vi "Create Session Reservation.vi"(7 "reservation observer":refnum<class "IReservation Observer.lvclass">, 8 "error in":errorcluster, 9 "session reservation response":T1, 10 "pin or relay names":string[](array[string]), 11 "pin map context":T8) -> (0 "error out":errorcluster, 3 "session reservation out":refnum<class "Session Reservation.lvclass">)   [LabVIEW 2020, in "Measurement Plugin Session Management V1.lvlib" / "Session Reservation.lvclass"]
doc: "Collects all the session reservation related data and creates a session reservation data value reference of the session reservation class."
uses:
  Session Reservation.lvclass
  gRPC/Generated APIs/ni/measurementlink/sessionmanagement/v1/RPC Messages/ni_measurementlink_PinMapContext.ctl
  IReservation Observer/IReservation Observer.lvclass
  gRPC/Generated APIs/ni/measurementlink/sessionmanagement/v1/RPC Messages/ni_measurementlink_sessionmanagement_v1_ReserveSessionsResponse.ctl
  gRPC/Generated APIs/ni/measurementlink/sessionmanagement/v1/RPC Messages/ni_measurementlink_sessionmanagement_v1_SessionInformation.ctl
  gRPC/Generated APIs/ni/measurementlink/sessionmanagement/v1/RPC Messages/nidevice_grpc_Session.ctl
  gRPC/Generated APIs/ni/measurementlink/sessionmanagement/v1/RPC Messages/ni_measurementlink_sessionmanagement_v1_ChannelMapping.ctl
  gRPC/Generated APIs/ni/measurementlink/sessionmanagement/v1/RPC Messages/ni_measurementlink_sessionmanagement_v1_MultiplexerSessionInformation.ctl
  gRPC/Generated APIs/ni/measurementlink/sessionmanagement/v1/RPC Messages/ni_measurementlink_sessionmanagement_v1_ReserveSessionsResponse_GroupMappingsEntry.ctl
  gRPC/Generated APIs/ni/measurementlink/sessionmanagement/v1/RPC Messages/ni_measurementlink_sessionmanagement_v1_ResolvedPinsOrRelays.ctl
  Data.ctl
  Session and Driver Info.ctl
  Sessions/Instrument Sessions/ISession Factory/ISession Factory.lvclass
  Sessions/Instrument Sessions/ISession Factory/Initialize and Close Session Behavior.ctl
  Connection Map/Connection Map.lvclass
  Group Mapping.ctl
  <vilib>/Utility/miscctls.llb/LVMapReplaceAction.ctl
  Session Reservation.lvclass/Session Reservation.ctl
  gRPC/Generated APIs/ni/measurementlink/sessionmanagement/v1/ni.measurementlink.sessionmanagement.v1.lvlib
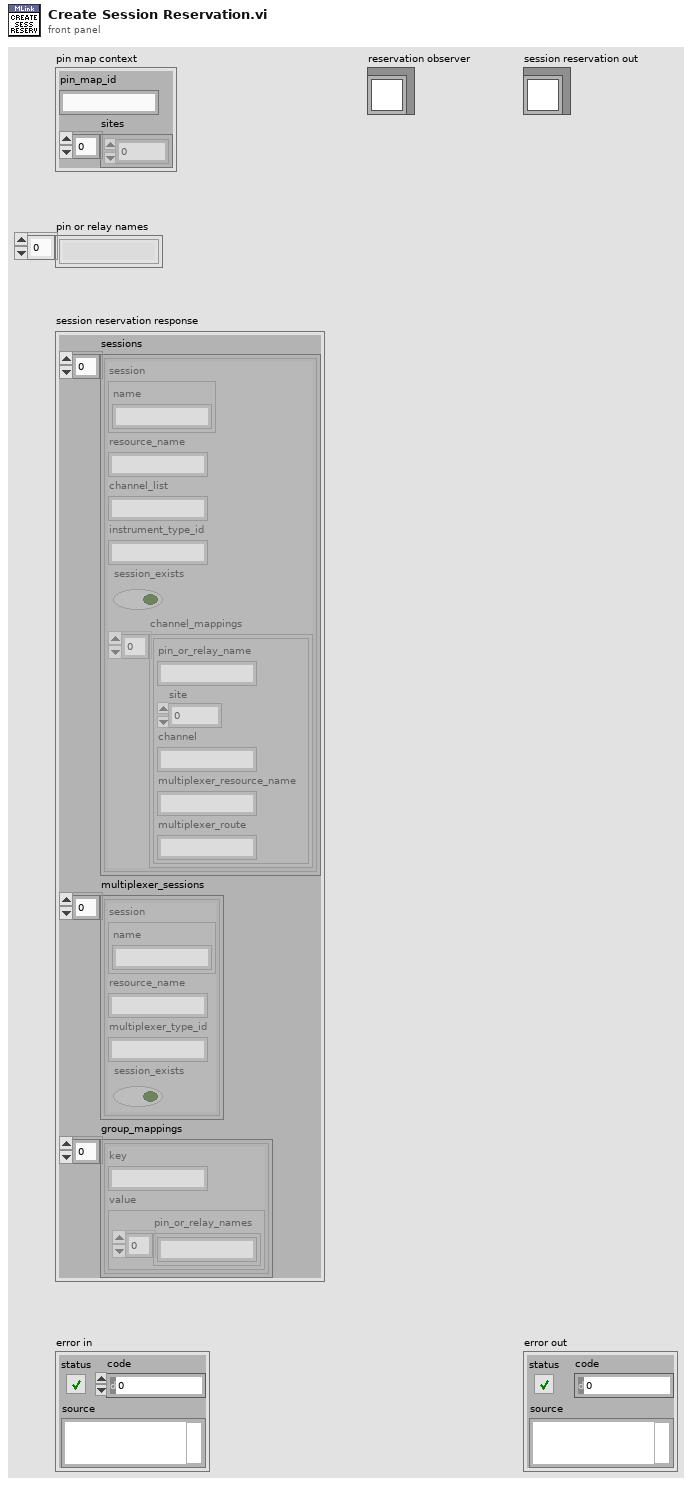
[diagram p1: front panel]
types:
  T1 = typedef "ni.measurementlink.sessionmanagement.v1.lvlib/ni_measurementlink_sessionmanagement_v1_ReserveSessionsResponse.ctl" = cluster{"sessions":T2[], "multiplexer_sessions":T5[], "group_mappings":T6[]}
  T2 = typedef "ni.measurementlink.sessionmanagement.v1.lvlib/ni_measurementlink_sessionmanagement_v1_SessionInformation.ctl" = cluster{"session":T3, "resource_name":string, "channel_list":string, "instrument_type_id":string, "session_exists":bool, "channel_mappings":T4[]}
  T3 = typedef "ni.measurementlink.sessionmanagement.v1.lvlib/nidevice_grpc_Session.ctl" = cluster{"name":string}
  T4 = typedef "ni.measurementlink.sessionmanagement.v1.lvlib/ni_measurementlink_sessionmanagement_v1_ChannelMapping.ctl" = cluster{"pin_or_relay_name":string, "site":i32, "channel":string, "multiplexer_resource_name":string, "multiplexer_route":string}
  T5 = typedef "ni.measurementlink.sessionmanagement.v1.lvlib/ni_measurementlink_sessionmanagement_v1_MultiplexerSessionInformation.ctl" = cluster{"session":T3, "resource_name":string, "multiplexer_type_id":string, "session_exists":bool}
  T6 = typedef "ni.measurementlink.sessionmanagement.v1.lvlib/ni_measurementlink_sessionmanagement_v1_ReserveSessionsResponse_GroupMappingsEntry.ctl" = cluster{"key":string, "value":T7}
  T7 = typedef "ni.measurementlink.sessionmanagement.v1.lvlib/ni_measurementlink_sessionmanagement_v1_ResolvedPinsOrRelays.ctl" = cluster{"pin_or_relay_names":string[]}
  T8 = typedef "ni.measurementlink.sessionmanagement.v1.lvlib/ni_measurementlink_PinMapContext.ctl" = cluster{"pin_map_id":string, "sites":i32[]}
  T9 = typedef "Measurement Plugin Session Management V1.lvlib/Session Reservation.lvclass/Data.ctl" = cluster{"session and driver infos":T10[], "pin or relay names":string[], "connection map":refnum<class "Connection Map.lvclass">, "pin map context":T8, "reservation observer":refnum<class "IReservation Observer.lvclass">, "dvr valid":bool, "group mappings":T12}
  T10 = typedef "Measurement Plugin Session Management V1.lvlib/Session Reservation.lvclass/Session and Driver Info.ctl" = cluster{"session info":T2, "session":variant, "session factory":refnum<class "ISession Factory.lvclass">, "initialize and close session behavior":T11}
  T11 = typedef "Instrument Sessions.lvlib/ISession Factory.lvclass/Initialize and Close Session Behavior.ctl" = enum16{"Initialize and Close", "Attach and Detach", "Initialize and Detach", "Attach and Close"}
  T12 = typedef "Measurement Plugin Session Management V1.lvlib/Session Reservation.lvclass/Group Mapping.ctl" = map{string, string[]}
  T13 = typedef "LVMapReplaceAction.ctl" = enum32{"Modify Entry only if found", "Add or Modify Entry", "Delete Entry"}
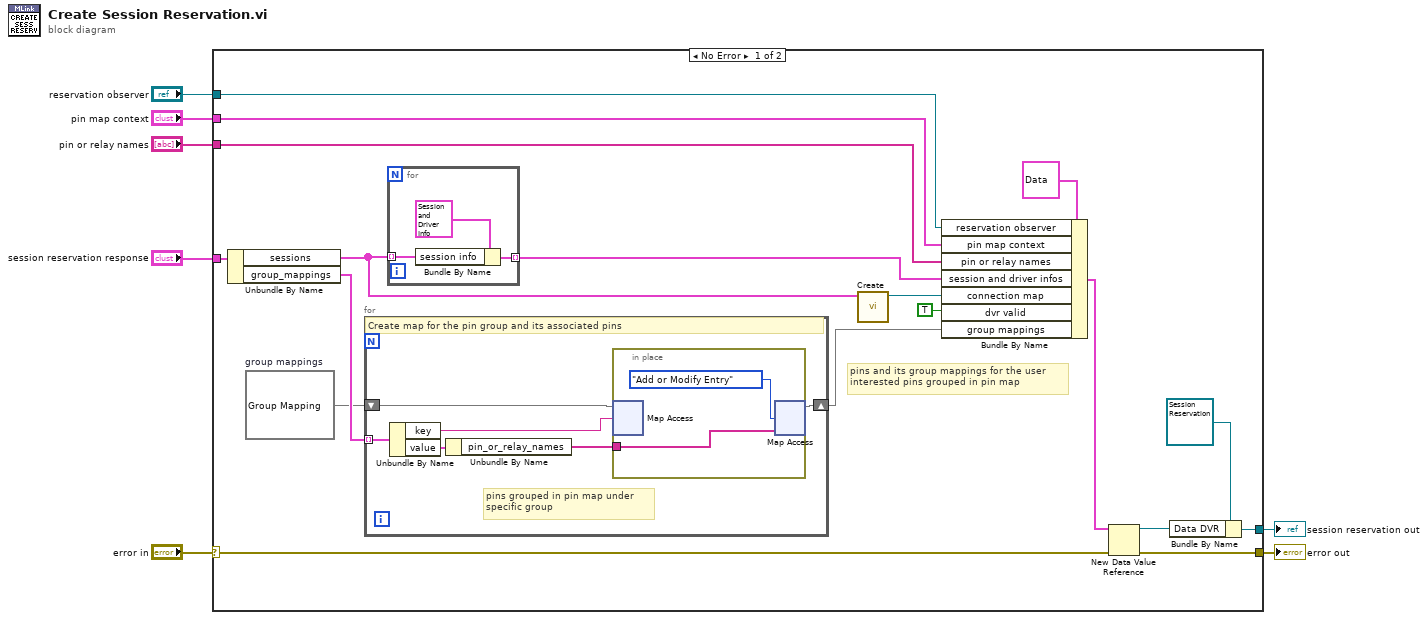
[diagram p0: block diagram]
diagram:
  n1 = case shown="No Error" "error in" {
    selector: "error in" -> [w15 w37]
    tunnel: [w19 w37] -> w7
    tunnel: [w18 _] -> w6
    tunnel: "pin map context" -> [w17 _]
    tunnel: "pin or relay names" -> [w16 _]
    tunnel: "reservation observer" -> [w14 _]
    tunnel: "session reservation response" -> [w12 _]
    frame No Error {
      w9 = T12 {}  # group mappings
      # "pins and its group mappings for the user \ninterested pins grouped in pin map"
      n2 = Unbundle By Name(w12) -> ("sessions"=w11:T2[], "group_mappings"=w10:T6[])
      n3 = for {
        tunnel: w10 -> [w31] mode=indexing
        shift-right: [w29] -> w8
        shift-left: w9 -> [w28]
        # "pins grouped in pin map under \nspecific group"
        # "Create map for the pin group and its associated pins"
        n4 = Unbundle By Name(w31) -> ("key"=w27:string, "value"=w30:T7)
        n5 = Unbundle By Name(w30) -> ("pin_or_relay_names"=w26:string[])
        n6 = in-place {
          in-place-border: w26 -> [w32]
          n7 = in-place-map #1(w28, w27) -> ()  [unwired: 1 in, 2 out]
          n8 = in-place-map #1(w32, LVMapReplaceAction."Add or Modify Entry" ("action")) -> (w29:T12)  [unwired: 2 out]
        }
      }
      n9 = for {
        tunnel: w11 -> [w36] mode=indexing
        tunnel: [w35] -> w25 mode=indexing
        n10 = Bundle By Name(cluster=T10 {"session info"={"session"={"name"=""}, "resource_name"="", "channel_list"="", "instrument_type_id"="", "session_exists"=FALSE, "channel_mappings"=[]}, "session"=variant, "session factory"=refnum, "initialize and close session behavior"=enum."Initialize and Close"} ("session and driver info"), "session info"=w36) -> (w35:T10)
      }
      n11 = call "Create.vi"("session info"=w11) -> ("connection map"=w24:refnum<class "Connection Map.lvclass">)  [unwired: 10 in]
      n12 = Bundle By Name(cluster=T9 {"session and driver infos"=[], "pin or relay names"=[], "connection map"=refnum, "pin map context"={"pin_map_id"="", "sites"=[]}, "reservation observer"=refnum, "dvr valid"=FALSE, "group mappings"={}} ("session reservation data"), "reservation observer"=w14, "pin map context"=w17, "pin or relay names"=w16, "session and driver infos"=w25, "connection map"=w24, "dvr valid"=TRUE, "group mappings"=w8) -> (w21:T9)
      n13 = New Data Value Reference(data value=w21, error in=w15) -> (data value reference=w23:refnum<data-value>, error out=w19:errorcluster)
      n14 = Bundle By Name(cluster=refnum<class "Session Reservation.lvclass"> refnum ("session reservation"), "Data DVR"=w23) -> (w18:refnum<class "Session Reservation.lvclass">)
    }
    frame Error {
    }
  }
  "error out" <- w7
  "session reservation out" <- w6
